vi "Find Ni-Scope digitizers.vi"(8 "Error In":errorcluster) -> (0 "Error Out":errorcluster, 2 "Device names out":string[](array[string]), 3 "Digitizers out":refnum<class "Pulse Driver.lvclass">[](array[class]))   [LabVIEW 2016, in "Ni-Scope Digitizer.lvclass"]
uses:
  Ni-Scope Digitizer.lvclass
  Instruments/Pulse Driver/Pulse Driver.lvclass
  C:/github/NHMFL_Core/Libraries/Instruments/Pulse Driver/Pulse Driver.lvclass
  NI-Scope Lock-in Driver/NI-Scope Lock-in Driver.lvclass
  C:/github/NHMFL_Core/Libraries/NI-DAQ/NI-Scope Digitizer/Ni-Scope Digitizer.lvclass
  C:/github/NHMFL_Core/Libraries/Instruments/Instrument Driver/Instrument Driver.lvclass
  Ni-Scope Digitizer.lvclass/Ni-Scope Digitizer.ctl
  Instruments/Instrument Driver/Instrument Driver.lvclass/Instrument Driver.ctl
  Write Device name.vi
  Instruments/Instrument Driver/Write Type ID.vi
  <instrlib>/niModInst/niModInst Get Installed Device Attribute (String).vi
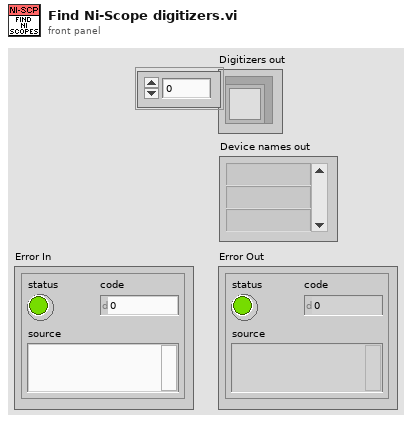
[diagram p1: front panel]
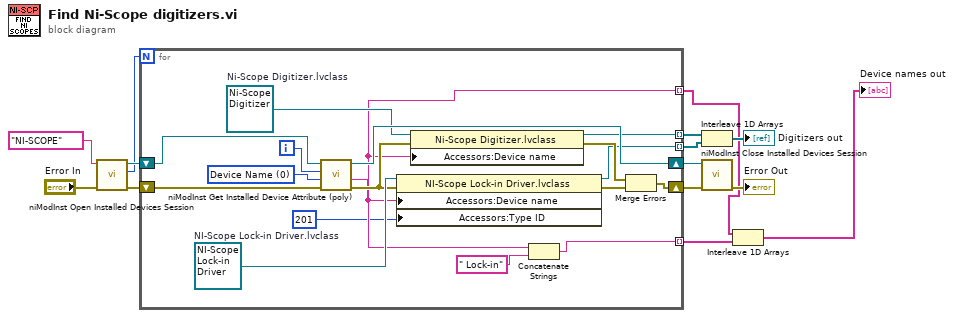
[diagram p0: block diagram]
diagram:
  n1 = call <instrlib>:"niModInst Open Installed Devices Session.vi"("error in (no error)"="Error In", "driver"="NI-SCOPE") -> ("error out"=w10:errorcluster, "device count"=w11:i32, "session"=w12:refnum<k20>)  [unwired: 7 in]
  n2 = for {
    N: w11 -> [_]
    shift-right: [w21] -> w8
    shift-left: w10 -> [w28]
    shift-right: [w29] -> w9
    shift-left: w12 -> [w30]
    tunnel: [w24] -> w6 mode=indexing
    tunnel: [w18] -> w3 mode=indexing
    tunnel: [w19] -> w4 mode=indexing
    tunnel: [w16] -> w2 mode=indexing
    i -> [w31]
    w23 = refnum<class "NI-Scope Lock-in Driver.lvclass"> refnum  # NI-Scope Lock-in Driver.lvclass
    w26 = refnum<class "Ni-Scope Digitizer.lvclass"> refnum  # Ni-Scope Digitizer.lvclass
    w27 = 0 items=["Device Name", "Device Model", "Serial Number"] ("attribute ID")
    n3 = call-poly <instrlib>:"niModInst Get Installed Device Attribute (poly).vi"("error in (no error)"=w28, "attribute ID"=w27, "index in"=w31, "session in"=w30) -> ("error out"=w22:errorcluster, "attribute value"=w18:string, "session out"=w29:refnum<k20>)  [unwired: 5 out]
    n4 = property class="NI-Scope Lock-in Driver.lvclass"(reference=w23, error in=w22, "Accessors:Device name"=w18, "Accessors:Type ID"=201 ("Type ID")) -> (reference out=w19:refnum<class "NI-Scope Lock-in Driver.lvclass">, error out=w20:errorcluster)
    n5 = property class="Ni-Scope Digitizer.lvclass"(reference=w26, error in=w22, "Accessors:Device name"=w18) -> (reference out=w24:refnum<class "Ni-Scope Digitizer.lvclass">, error out=w25:errorcluster)
    n6 = Concatenate Strings(w18, " Lock-in" ("string")) -> (w16:string)
    n7 = Merge Errors(w25, w20) -> (w21:errorcluster)
  }
  n8 = Interleave 1D Arrays(w6, w4) -> (→"Digitizers out":refnum<class "Ni-Scope Digitizer.lvclass">[])
  n9 = call <instrlib>:"niModInst Close Installed Devices Session.vi"("error in (no error)"=w8, "session"=w9) -> ("error out"=→"Error Out":errorcluster)  [unwired: 9 out]
  n10 = Interleave 1D Arrays(w3, w2) -> (→"Device names out":string[])
